vi "Constants.vi"() -> ()   [LabVIEW 2020, in "G5 Regatron Custom Device Shared.lvlib"]
doc: "Use this Global VI to access the GUIDs assigned to the page resources of the Custom Device."
uses:
  G5 Regatron Custom Device Shared.lvlib
panel:
  in  "Tab Control":enum32{"GUIDs", "Constants", "Properties"}(tab)
  in  "G5 Regatron Custom Device":string="53720824-6858-4655-a7de-cc71540320c5"
  in  "IP.Address":string="Compiled.Settings"
  in  "Compiled.Settings":string="Compiled.Settings"
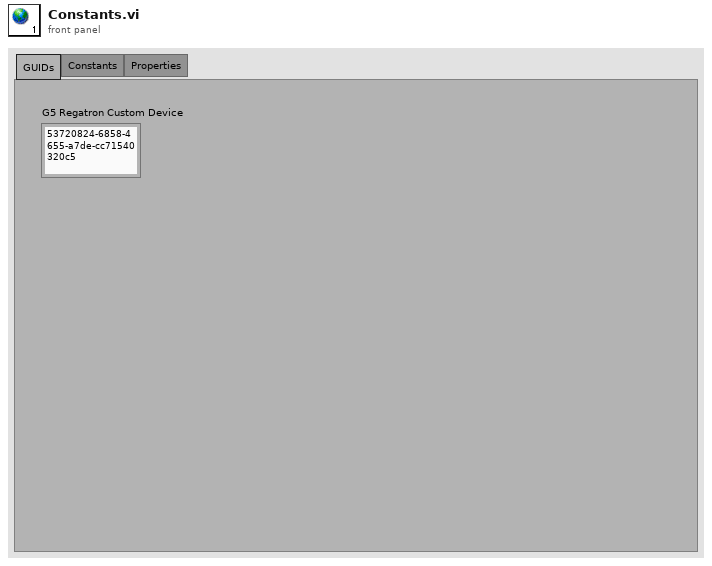
[diagram p1: front panel]
diagram:
